vi "gauss.vi"(6 "AA":dbl, 7 "ys":dbl, 9 "xs":dbl, 10 "R":dbl, 11 "field":T1) -> (3 "field out":T1)   [LabVIEW 2012, in "LightPipes.lvlib"]
doc: "__declspec(dllexport) void gauss(FIELD* field, double R, double xs, double ys, double AA );"
uses:
  LightPipes.lvlib
  Lightpipes.dll
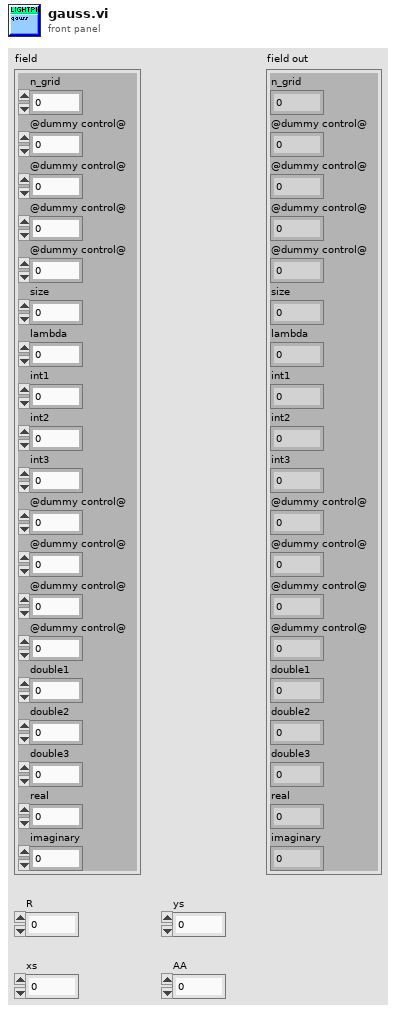
[diagram p1: front panel]
types:
  T1 = cluster{"n_grid":i32, "@dummy control@":i8, "@dummy control@":i8, "@dummy control@":i8, "@dummy control@":i8, "size":dbl, "lambda":dbl, "int1":i32, "int2":i32, "int3":i32, "@dummy control@":i8, "@dummy control@":i8, "@dummy control@":i8, "@dummy control@":i8, "double1":dbl, "double2":dbl, "double3":dbl, "real":u32, "imaginary":u32}
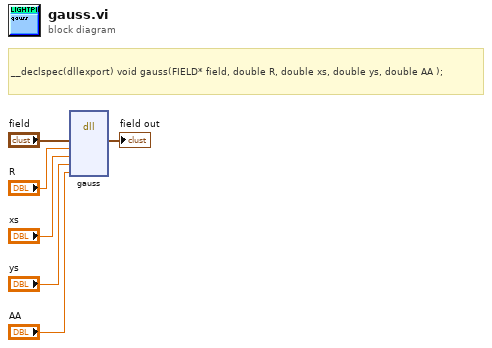
[diagram p0: block diagram]
diagram:
  # "__declspec(dllexport) void gauss(FIELD* field, double R, double xs, double ys, double AA );"
  n1 = dll-call lib="C:/Users/Tri/Documents/Gerchberg/LightPipes.*" fn="gauss"("field"="field", "R"="R", "xs"="xs", "ys"="ys", "AA"="AA") -> ("field"=→"field out":T1)  [unwired: 8 in, 2 out]
